vi "Recombined&noise.vi"(6 "right":i16, 7 "Input 3":u8[][](array[numeric]), 9 "bottom":i16, 10 "input 2":u8[][](array[numeric]), 11 "Inpupt":u8[][](array[numeric])) -> (2 "Rectangle.right":i16, 3 "Rectangle.bottom":i16, 4 "new picture":picture, 5 "output image array":u8[](array[numeric]))   [LabVIEW 2016]
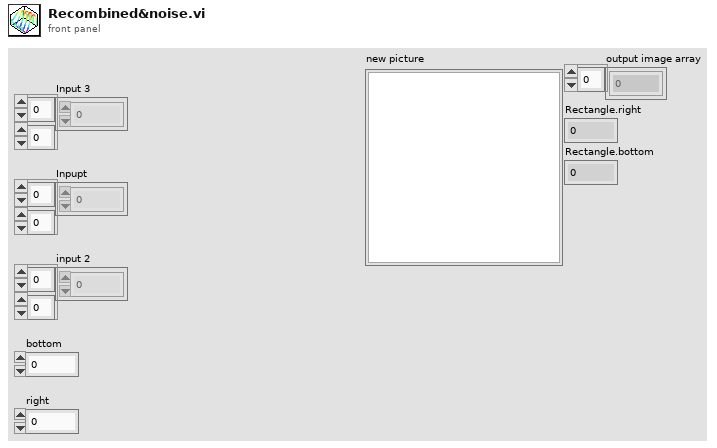
[diagram p1: front panel]
types:
  T1 = typedef "imagedata.ctl" = cluster{"image type":i32, "image depth":i32, "image":u8[], "mask":u8[], "colors":u32[], "Rectangle":cluster{"left":i16, "top":i16, "right":i16, "bottom":i16}}
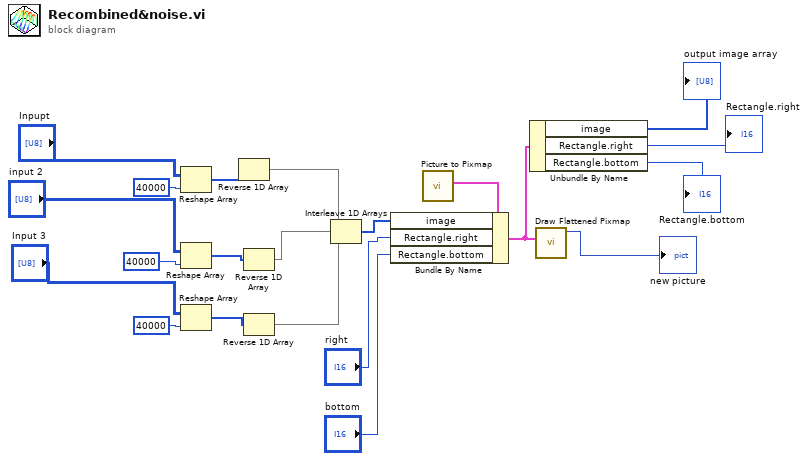
[diagram p0: block diagram]
diagram:
  n1 = Reshape Array("Inpupt", 40000 ("dimension size")) -> (w12:u8[])
  n2 = Reshape Array("input 2", 40000 ("dimension size")) -> (w14:u8[])
  n3 = Reshape Array("Input 3", 40000 ("dimension size")) -> (w16:u8[])
  n4 = Reverse 1D Array(array=w12) -> (reversed array=w13:u8[])
  n5 = Reverse 1D Array(array=w14) -> (reversed array=w15:u8[])
  n6 = Reverse 1D Array(array=w16) -> (reversed array=w17:u8[])
  n7 = Interleave 1D Arrays(w13, w15, w17) -> (w1:u8[])
  n8 = call <vilib>:"Picture to Pixmap.vi"() -> ("image data"=w20:T1)  [unwired: 10 in, 1 out]
  n9 = Bundle By Name(cluster=w20, "image"=w1, "Rectangle.right"="right", "Rectangle.bottom"="bottom") -> (w5:T1)
  n10 = Unbundle By Name(w5) -> ("image"=→"output image array":u8[], "Rectangle.right"=→"Rectangle.right":i16, "Rectangle.bottom"=→"Rectangle.bottom":i16)
  n11 = call <vilib>:"Draw Flattened Pixmap.vi"("image data"=w5) -> ("new picture"=→"new picture":picture)  [unwired: 8 in]
